vi "Next Action.vi"(11 "Action Stack":string) -> (1 "Action's Argument":string, 2 "Next Action (top of stack)":string, 3 "Remaining Actions":string)   [LabVIEW 2020, in "Action Stack.lvlib"]
doc: "Parses the Action Stack and returns the next action with the associated arguments.\n\nThis provides the functionality of the JKI Statemachine \"Parse State Queue\" vi, but without the error input.\n\n<B>Action Syntax:</B>\nAction >> Argument\nAction separator: Line feed\nTo add a comment use \"//\" or \"#\" and all text to the right will be ignored\n\n<B>Example:</B>\n//Initial Actions\nUI:Initialize // This initializes the UI\nData:Initialize\nUpdate >> Full // initial update of everything"
uses:
  <vilib>/JDP Science/JDP Science Common Utilities/Action Stack/Action Stack.lvlib
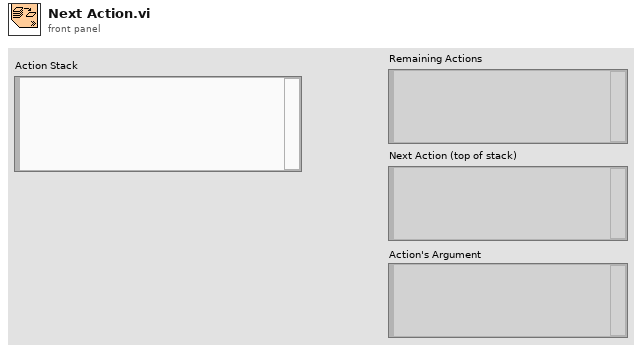
[diagram p1: front panel]
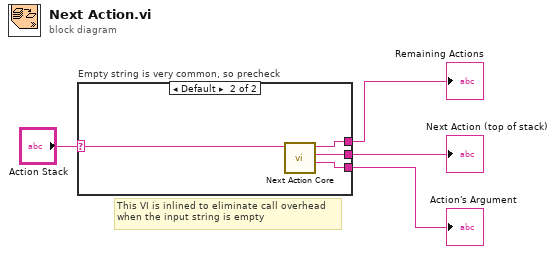
[diagram p0: block diagram]
diagram:
  # "This VI is inlined to eliminate call overhead\nwhen the input string is empty"
  n1 = case "Empty string is very common, so precheck" shown="Default" "Action Stack" {
    selector: "Action Stack" -> [w5 w9]
    tunnel: [_ w8] -> w4
    tunnel: [w5 w7] -> w3
    tunnel: [_ w6] -> w2
    frame "" {
    }
    frame Default {
      n2 = call <vilib>:"Next Action Core.vi"("Actions"=w9) -> ("Arguments"=w6:string, "Next Action"=w7:string, "Remaining Actions"=w8:string)  [unwired: 8 in]
    }
  }
  "Remaining Actions" <- w4
  "Next Action (top of stack)" <- w3
  "Action's Argument" <- w2
